vi "ExtendedKalmanFilter_GetXHat_Single.vi"(10 "Row":i32, 11 "in ExtendedKalmanFiilter":T1) -> (3 "xHat Value":dbl)   [LabVIEW 2019, in "Trajectory_Library.lvlib"]
doc: "Returns an element of the state estimate x-hat.\n \nInputs:\n - inExtendedKalmanFIlter -- filter data cluster\n - row Row of x-hat.\n\nReturns:\n - xHat_value -- the value of the state estimate x-hat at i."
uses:
  Trajectory_Library.lvlib
  TypeDef/EXTENDED_KALMAN_FILTER.ctl
  <vilib>/Analysis/Matrix/Datatypes/RealMatrix.ctl
  <vilib>/Analysis/Matrix/NI_Matrix.lvlib
panel:
  # "State Estimate <Statess,1>"
  # "<States, States>"
  # "<States, States>"
  # "<Statess,  States>"
  # "<Outputs, Outputs>"
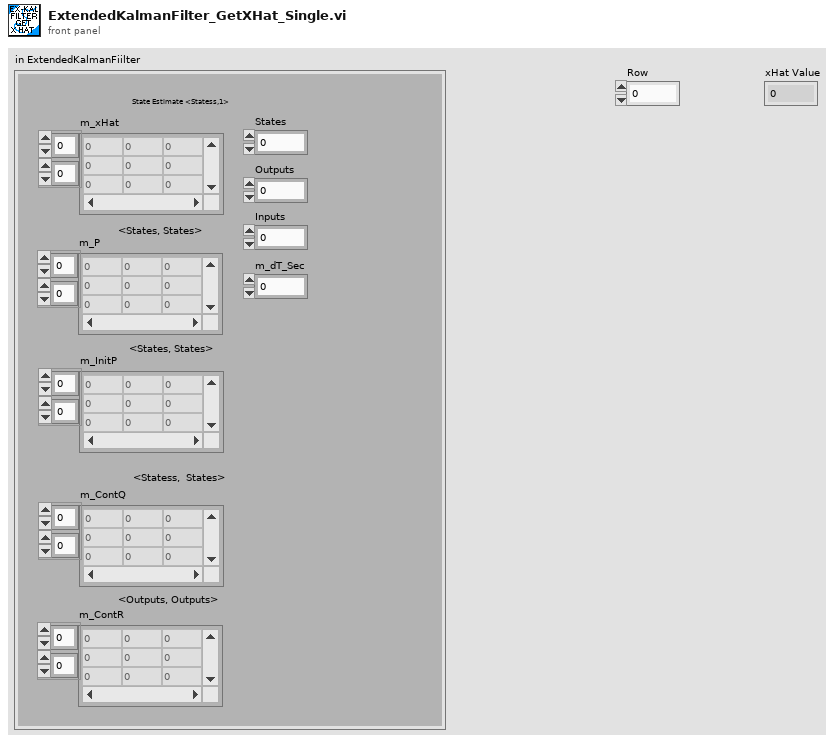
[diagram p1: front panel]
types:
  T1 = typedef "Trajectory_Library.lvlib/EXTENDED_KALMAN_FILTER.ctl" = cluster{"m_P":T2, "m_xHat":T2, "States":i32, "Outputs":i32, "m_ContR":T2, "m_ContQ":T2, "m_dT_Sec":dbl, "Inputs":i32, "m_InitP":T2}
  T2 = typedef "NI_Matrix.lvlib/RealMatrix.ctl" = dbl[][]
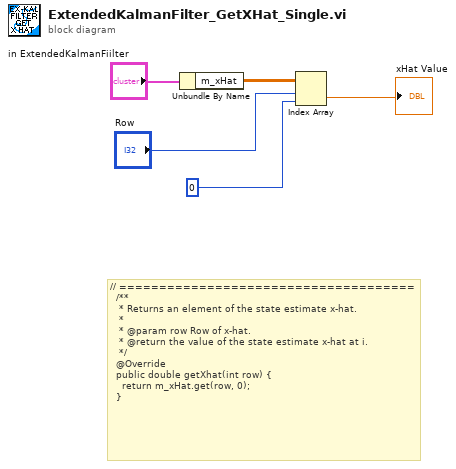
[diagram p0: block diagram]
diagram:
  # "// =====================================\n  /**\n   * Returns an element of the state estimate x-hat.\n   *\n   * @param row Row of x-hat.\n   * @return the value of the state estimate x-hat at i.\n   */\n  @Override\n  public double getXhat(int row) {\n    return m_xHat.get(row, 0);\n  }"
  n1 = Unbundle By Name("in ExtendedKalmanFiilter") -> ("m_xHat"=w5:T2)
  n2 = Index Array(array=w5, index (row)="Row", index (col)=0) -> (element=→"xHat Value":dbl)
